vi "AdaptToInputs.vi"(3 "Term Types":T1[](array[typedef]), 4 "XRef":refnum<vi>, 5 "State In":T4={"Input Type"=variant(dbl 0.0), "Selection"=0, "Element Names"=[], "Type Strings"=[], "Element Types"=[]}) -> (0 "Reply":string[](array[string]), 2 "State Out":T4={"Input Type"=variant(dbl 0.0), "Selection"=0, "Element Names"=[], "Type Strings"=[], "Element Types"=[]})   [LabVIEW 2015, in "Construct-Tagged-Union.xnode"]
doc: "This ability VI is called by LabVIEW during type propagation so that your XNode may adapt itself to new input types. Term Types is an array of pairs of current Term IDs and the type descriptors corresponding to them. The type descriptors are taken from the signal connected to the terminal. Unwired terminals are not included in the array. Use Reply to inform LabVIEW of any actions it needs to take.\n\nDefault behavior: None.\n\nThis ability does not provide UI and OS messages are not handled."
uses:
  Construct-Tagged-Union.xnode
  State.ctl
  <vilib>/XNodeSupport/XNodeTermTypeIDPair.ctl
  <vilib>/XNodeSupport/XNodeType.ctl
  <vilib>/XNodeSupport/XNodeString.ctl
  <vilib>/Erdos Miller/LV-Scripting/LV-Scripting.lvlib
  <vilib>/Utility/Data Type/NI_Data Type.lvlib
  <vilib>/XNodeSupport/NI_XNodeSupport.lvlib
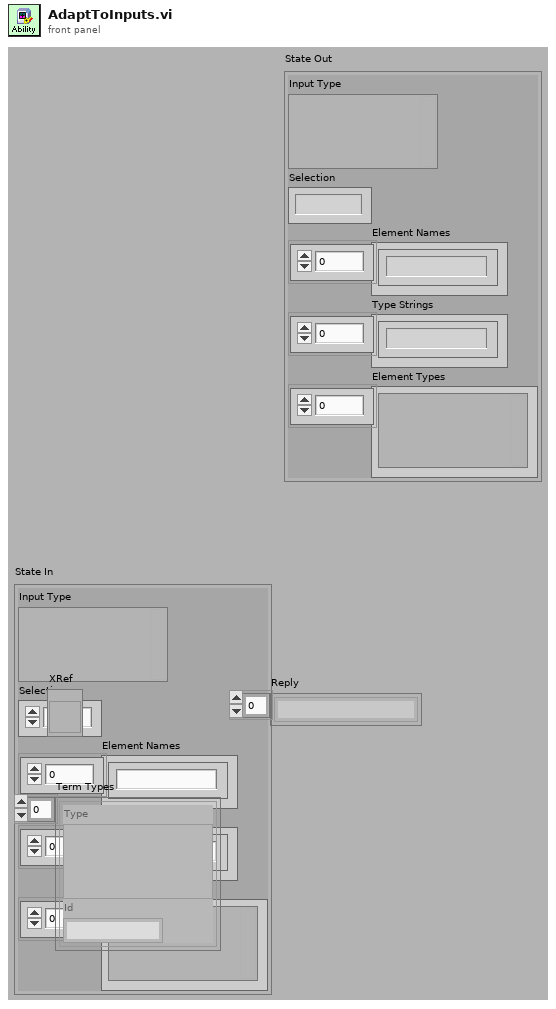
[diagram p1: front panel]
types:
  T1 = typedef "NI_XNodeSupport.lvlib/XNodeTermTypeIDPair.ctl" = cluster{"Type":T2, "Id":T3}
  T2 = typedef "NI_XNodeSupport.lvlib/XNodeType.ctl" = variant
  T3 = typedef "NI_XNodeSupport.lvlib/XNodeString.ctl" = string
  T4 = typedef "Construct-Tagged-Union.xnode/State.ctl" = cluster{"Input Type":variant, "Selection":i32, "Element Names":string[], "Type Strings":string[], "Element Types":variant[]}
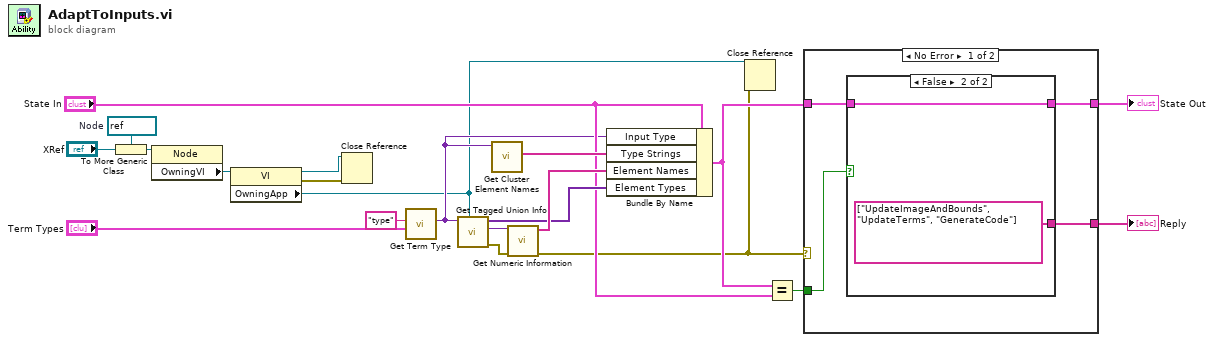
[diagram p0: block diagram]
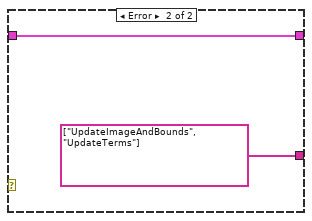
[diagram p3: hidden frame]
diagram:
  w7 = refnum<vi> refnum  # Node
  n1 = To More Generic Class(target class=w7, reference="XRef") -> (generic class reference=w6:refnum<vi>)
  n2 = property class="Node"(reference=w6) -> ("OwningVI"=w5:refnum<vi>)  [unwired: 1 in, 2 out]
  n3 = property class="VI"(reference=w5) -> (reference out=w4:refnum<vi>, error out=w3:errorcluster, "OwningApp"=w2:refnum<vi>)  [unwired: 1 in]
  n4 = Close Reference(reference=w4, error in (no error)=w3) -> ()  [unwired: 1 out]
  n5 = call <vilib>:"Get Term Type.vi"("Term Types"="Term Types", "ID"="type") -> ("Type"=w9:variant)  [unwired: 9 in]
  n6 = call <vilib>:"Get Tagged Union Info.vi"("application reference (local)"=w2, "Type in"=w9) -> ("error out"=w17:errorcluster, "Enum Type"=w15:variant, "Element Types"=w13:variant[])  [unwired: 7 in]
  n7 = call <vilib>:"Get Cluster Element Names.vi"("Cluster in"=w9) -> ("Names"=w16:string[])  [unwired: 8 in, 2 out]
  n8 = call <vilib>:"Get Numeric Information.vi"("error in (no error)"=w17, "Variant"=w15) -> ("error out"=w1:errorcluster, "Enum Names"=w14:string[])  [unwired: 6 in, 2 out]
  n9 = Bundle By Name(cluster="State In", "Input Type"=w9, "Type Strings"=w16, "Element Names"=w14, "Element Types"=w13) -> (w10:T4)
  n10 = Close Reference(reference=w2, error in (no error)=w1) -> ()  [unwired: 1 out]
  n11 = Equal?(x=w10, y="State In") -> (x = y?=w12:bool)
  n12 = case shown="No Error" w1 {
    tunnel: [w25 string[] ["UpdateImageAndBounds", "UpdateTerms"] ("Reply")] -> w19
    tunnel: w10 -> [w23 w30]
    tunnel: [w24 w30] -> w18
    tunnel: w12 -> [w22 _]
    frame No Error {
      n13 = case shown="False" w22 {
        tunnel: [_ string[] ["UpdateImageAndBounds", "UpdateTerms", "GenerateCode"] ("Reply")] -> w25
        tunnel: w23 -> [w26 w27]
        tunnel: [w26 w27] -> w24
        frame True {
        }
        frame False {
        }
      }
    }
    frame Error {
    }
  }
  "Reply" <- w19
  "State Out" <- w18
